vi "Generate Event.vi"(4 "Error In":errorcluster) -> (0 "Error Out":errorcluster)   [LabVIEW 2015, in "ude_Stop Application.lvlib"]
uses:
  ude_Stop Application.lvlib
  Event Data.ctl
panel:
  in  "event data":T1
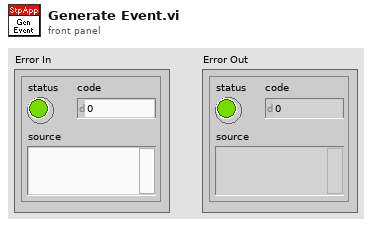
[diagram p1: front panel]
types:
  T1 = typedef "ude_Stop Application.lvlib/Event Data.ctl" = variant
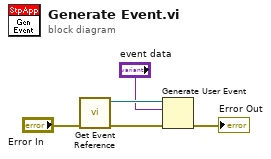
[diagram p0: block diagram]
diagram:
  n1 = call "Get Event Reference.vi"("error in (no error)"="Error In") -> ("error out"=w4:errorcluster, "Stop Application"=w3:refnum<user-event>)  [unwired: 5 in]
  n2 = Generate User Event(user event=w3, event data cluster="event data", error in=w4) -> (error out=→"Error Out":errorcluster)  [unwired: 1 in, 1 out]
